vi "integrate energy.vi"(8 "ellipse fit":T3, 9 "pulse statistics":T2, 10 "crossing stats":T4, 11 "integration cluster":T1) -> (0 "elapsed time":dbl, 1 "half cycles counted":dbl, 3 "integration cluster out":T1)   [LabVIEW 2017]
uses:
  typedefs/magnetic field fit.ctl
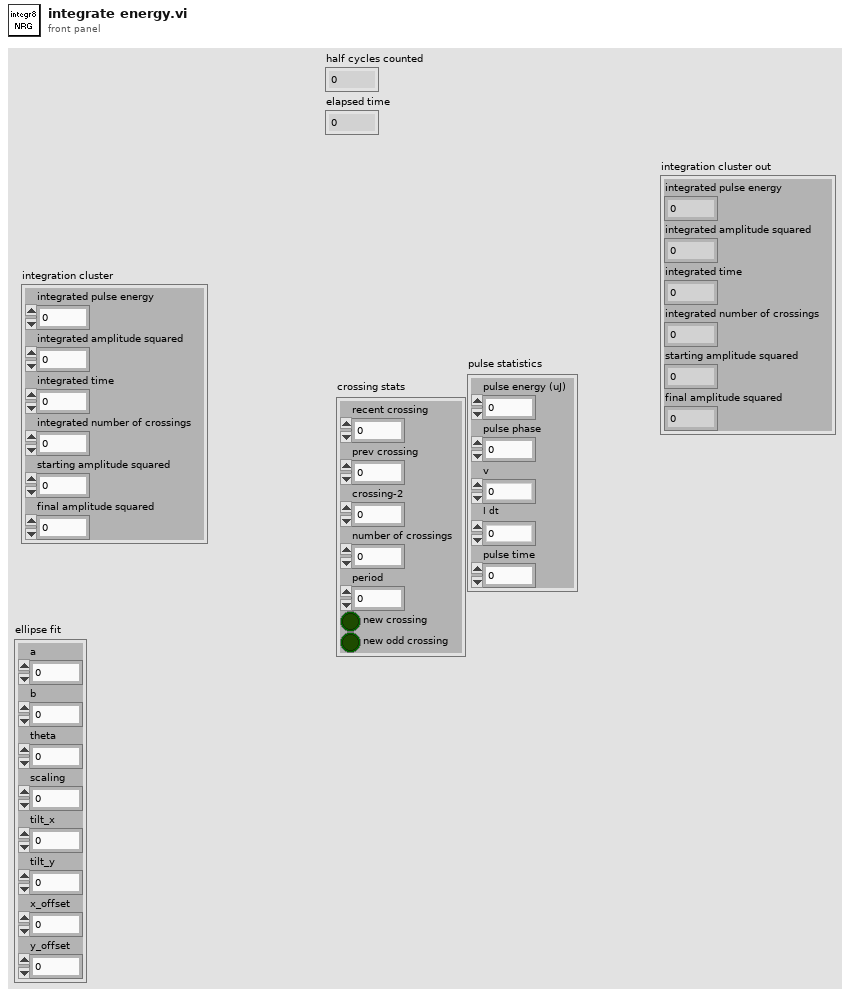
[diagram p1: front panel]
types:
  T1 = cluster{"integrated pulse energy":dbl, "integrated amplitude squared":dbl, "integrated time":dbl, "integrated number of crossings":dbl, "starting amplitude squared":dbl, "final amplitude squared":dbl}
  T2 = cluster{"pulse energy (uJ)":sgl, "pulse phase":dbl, "v":dbl, "I dt":dbl, "pulse time":dbl}
  T3 = typedef "magnetic field fit.ctl" = cluster{"a":dbl, "b":dbl, "theta":dbl, "scaling":dbl, "tilt_x":dbl, "tilt_y":dbl, "bx_offset":dbl, "by_offset":dbl, "bz_offset":dbl, "x_offset":dbl, "y_offset":dbl}
  T4 = cluster{"recent crossing":dbl, "prev crossing":dbl, "crossing-2":dbl, "number of crossings":i32, "period":dbl, "new crossing":bool, "new odd crossing":bool}
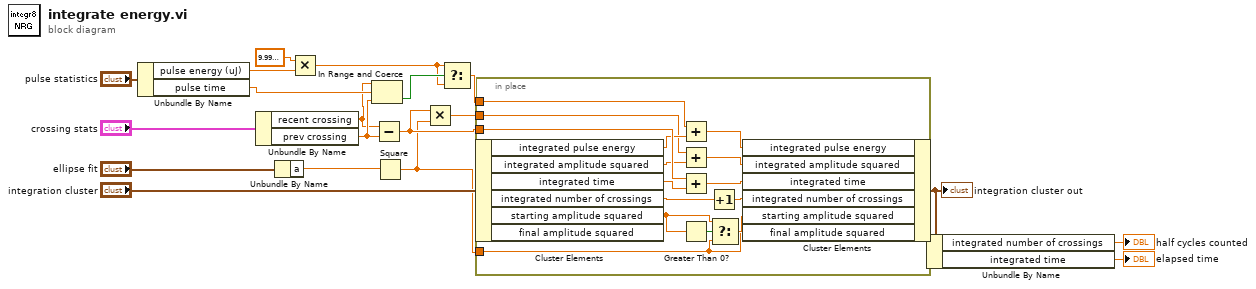
[diagram p0: block diagram]
diagram:
  n1 = Unbundle By Name("pulse statistics") -> ("pulse energy (uJ)"=w16:sgl, "pulse time"=w7:dbl)
  n2 = Unbundle By Name("crossing stats") -> ("recent crossing"=w5:dbl, "prev crossing"=w6:dbl)
  n3 = Unbundle By Name("ellipse fit") -> ("a"=w14:dbl)
  n4 = Multiply(x=sgl 1e-06, y=w16) -> (x*y=w1:sgl)
  n5 = In Range and Coerce(upper limit=w5, x=w7, lower limit=w6) -> (In Range?=w9:bool)  [unwired: 1 out]
  n6 = Subtract(x=w5, y=w6) -> (x-y=w13:dbl)
  n7 = Square(x=w14) -> (x^2=w11:dbl)
  n8 = Multiply(x=w13, y=w11) -> (x*y=w12:dbl)
  n9 = Select(t=w1, s=w9, f=w1) -> (s? t:f=w8:sgl)
  n10 = in-place {
    in-place-border: w13 -> [w33]
    in-place-border: w8 -> [w31]
    in-place-border: w12 -> [w27]
    in-place-border: w11 -> [w20]
    n11 = in-place-cluster #1("integration cluster") -> ("integrated pulse energy"=w32:dbl, "integrated amplitude squared"=w28:dbl, "integrated time"=w34:dbl, "integrated number of crossings"=w30:dbl, "starting amplitude squared"=w22:dbl)  [unwired: 1 out]
    n12 = Add(x=w31, y=w32) -> (x+y=w26:dbl)
    n13 = Add(x=w27, y=w28) -> (x+y=w25:dbl)
    n14 = Add(x=w33, y=w34) -> (x+y=w24:dbl)
    n15 = Greater Than 0?(x=w22) -> (x > 0?=w23:bool)
    n16 = Increment(x=w30) -> (x+1=w29:dbl)
    n17 = Select(t=w22, s=w23, f=w20) -> (s? t:f=w21:dbl)
    n18 = in-place-cluster #1("integrated pulse energy"=w26, "integrated amplitude squared"=w25, "integrated time"=w24, "integrated number of crossings"=w29, "starting amplitude squared"=w21, "final amplitude squared"=w20) -> (w4:T1)
  }
  "integration cluster out" <- w4
  n19 = Unbundle By Name(w4) -> ("integrated number of crossings"=→"half cycles counted":dbl, "integrated time"=→"elapsed time":dbl)
